vi "S Parameter VST Measurement.vi"(8 "error in":errorcluster, 9 "SPML Settings":T2={"VST Resource Name"="5842_0", "RFSG Port"="Port1", "RFmx Port"="Port2", "RF Out Switch"="2599_S8", "RF Out Connection"={"Common RFout"="COM0", "Port1 Incident"="NC0", "Port2 Incident"="NO0"}, "RF In Switch"="2597_S12", "RF In Connection"={"Common RFin"="COM", "Port1 Reference"="CH1", "Port1 Test"="CH2", "Port2 Reference"="CH4", "Port2 Test"="CH3"}, "RFSG attenuation mode"=enum."<None>", "RFSG Constant Attenuation (dB)"=0.0, "Save Calibration File at"=path "", "Short S1P"=path "", "Open S1P"=path "", "Load S1P"=path "", "Through Adapter S2P"=path ""}, 11 "Test Configuration":T1={"Action"=enum."Measure", "Power Level (dBm)"=0.0, "External Gain (dB)"=-6.0, "Frequency Sweep"={"Start Frequency (Hz)"=6000000000.0, "Stop Frequency (Hz)"=12000000000.0, "Step Size (Hz)"=100000000.0}, "Type of Stimulus"=enum."CW", "Pulse Width (s)"=0.0, "PRI (s)"=0.0, "IF Bandwidth (Hz)"=10000.0, "Average Mode"=enum."Per Sweep", "Number of Averages"=1, "SnP File Path"=path "", "Calibration File Path"=path "C:/Users/ies-pg-8881/Desktop/Andy/FPT/S_param_VST/S_param_cal_4.tdms"} {"Frequency Sweep"."Step Size (Hz)" format="%#_6p"; "Frequency Sweep"."Stop Frequency (Hz)" format="%.3p"; "Frequency Sweep"."Start Frequency (Hz)" format="%.3p"}) -> (0 "error out":errorcluster={"status"=TRUE, "code"=-1074134944, "source"="RFmxVNA Calibration Initiate.vi\r\n<ERR>IVI: (Hex 0xBFFA0060) Insufficient location information or resource not present in the system.  "}, 5 "S-Param Phase":dbl[][](array[numeric]), 7 "S-Param Magnitude":dbl[][](array[numeric]))   [LabVIEW 2023]
uses:
  Controls/Hardware Config - SParam_VST.ctl
  Controls/Test Config - SParam_VST.ctl
  <vilib>/niSPML/S-Parameter Measurements.lvlib
panel:
  out "SParam3":T3(graph)
  out "SParam1":T3(graph)
  out "SParam2":T3(graph)
  out "SParam0":T3(graph)
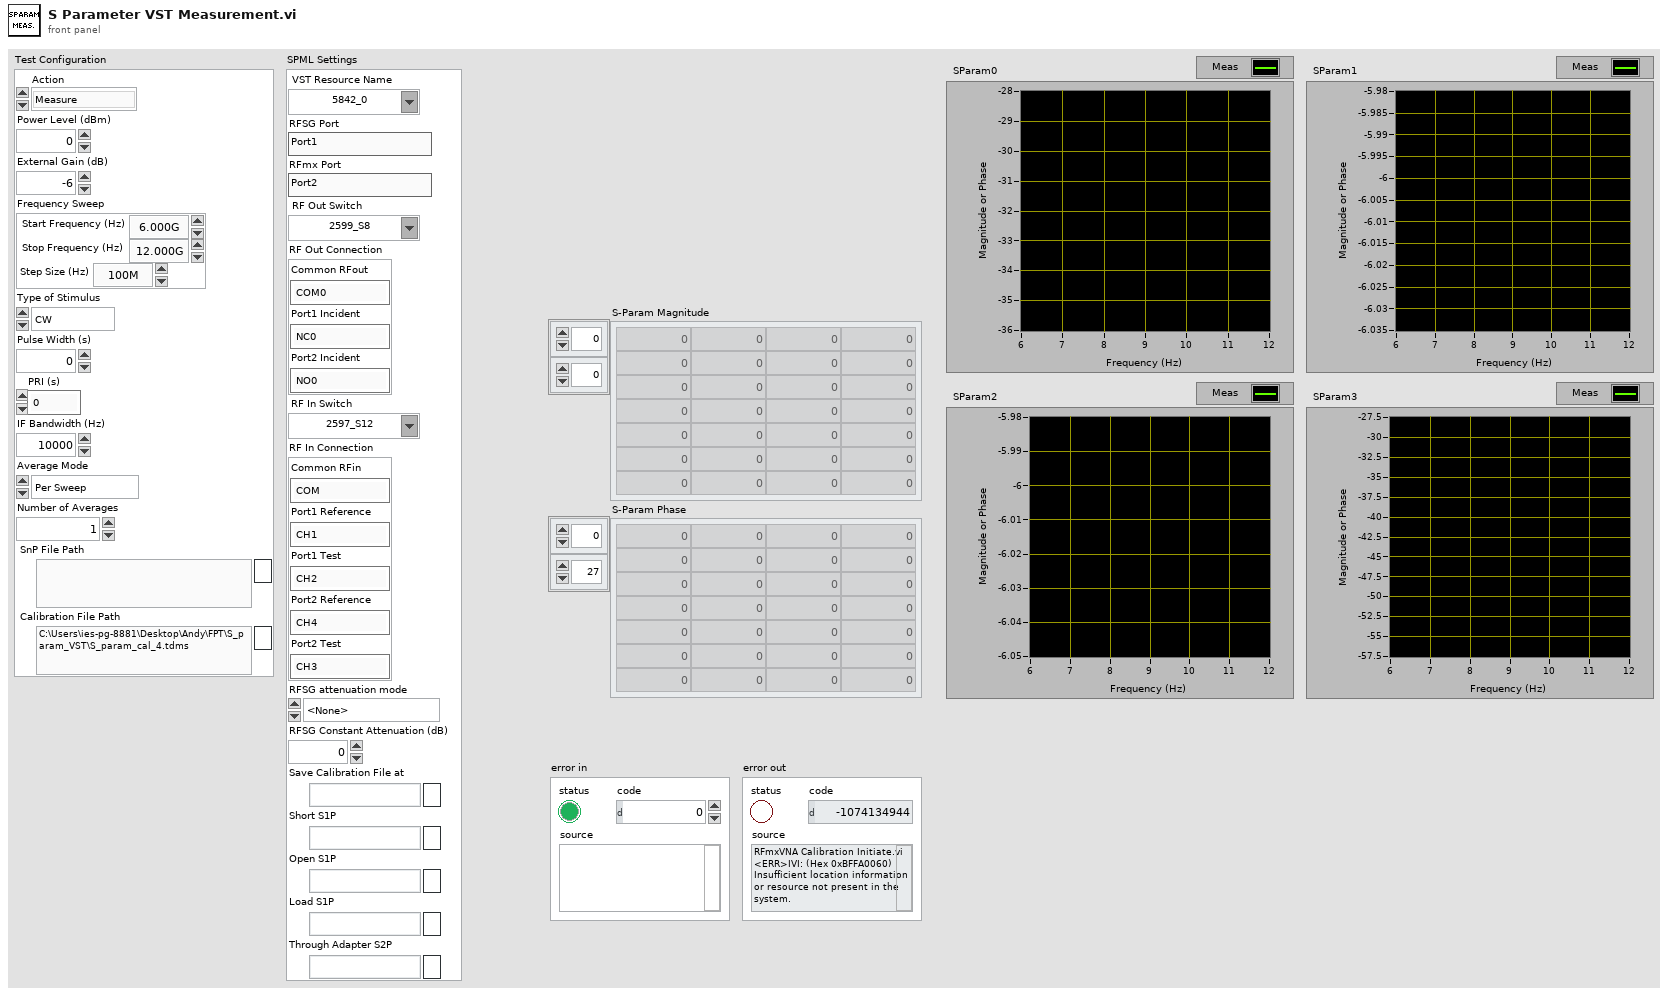
[diagram p1: front panel]
types:
  T1 = typedef "Test Config - SParam_VST.ctl" = cluster{"Action":enum32{"Calibrate", "Measure"}, "Power Level (dBm)":dbl, "External Gain (dB)":dbl, "Frequency Sweep":cluster{"Start Frequency (Hz)":dbl, "Stop Frequency (Hz)":dbl, "Step Size (Hz)":dbl}, "Type of Stimulus":enum16{"CW", "Pulsed CW"}, "Pulse Width (s)":dbl, "PRI (s)":dbl, "IF Bandwidth (Hz)":dbl, "Average Mode":enum16{"Per Sweep", "Per Point"}, "Number of Averages":i32, "SnP File Path":path, "Calibration File Path":path}
  T2 = typedef "Hardware Config - SParam_VST.ctl" = cluster{"VST Resource Name":refnum<k15>, "RFSG Port":string, "RFmx Port":string, "RF Out Switch":refnum<k15>, "RF Out Connection":cluster{"Common RFout":string, "Port1 Incident":string, "Port2 Incident":string}, "RF In Switch":refnum<k15>, "RF In Connection":cluster{"Common RFin":string, "Port1 Reference":string, "Port1 Test":string, "Port2 Reference":string, "Port2 Test":string}, "RFSG attenuation mode":enum32{"<None>", "Constant Attenuation"}, "RFSG Constant Attenuation (dB)":dbl, "Save Calibration File at":path, "Short S1P":path, "Open S1P":path, "Load S1P":path, "Through Adapter S2P":path}
  T3 = cluster{"S-Param Magnitude":dbl[], "S-Param Magnitude":dbl[]}
  T4 = typedef "S-Parameter Measurements.lvlib/S-Par Reference.lvclass/Session Handle.ctl" = refnum<data-value>
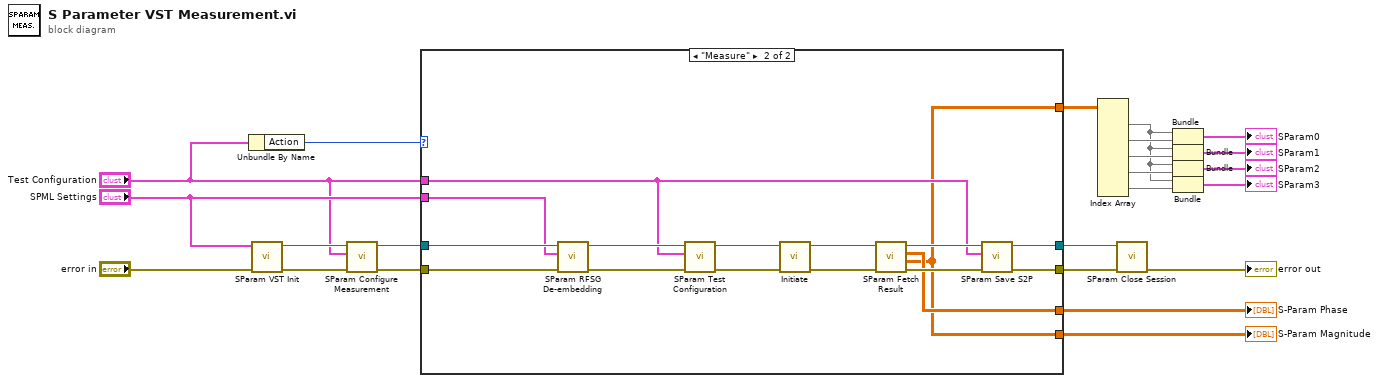
[diagram p0: block diagram]
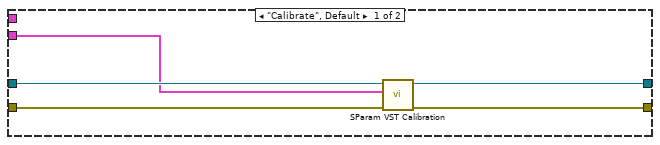
[diagram p2: hidden frame]
diagram:
  n1 = Unbundle By Name("Test Configuration") -> ("Action"=w22:enum32{"Calibrate", "Measure"})
  n2 = call "SParam VST Init.vi"("error in"="error in", "SPML Settings"="SPML Settings") -> ("error out"=w18:errorcluster, "S-Par Reference Out"=w17:T4)  [unwired: 8 in]
  n3 = call "SParam Configure Measurement.vi"("error in"=w18, "Test Configuration"="Test Configuration", "S-Par Reference In"=w17) -> ("error out"=w14:errorcluster, "S-Par Reference Out"=w15:T4)  [unwired: 7 in]
  n4 = case shown="\"Measure\"" w22 {
    tunnel: [_ w29] -> w13
    tunnel: [w25 w35] -> w3
    tunnel: [w24 w44] -> w2
    tunnel: w15 -> [w27 w40]
    tunnel: w14 -> [w28 w41]
    tunnel: "Test Configuration" -> [_ w31]
    tunnel: "SPML Settings" -> [w26 w32]
    tunnel: [_ w29] -> w21
    tunnel: [_ w30] -> w20
    frame "Calibrate", Default {
      n5 = call "SParam VST Calibration.vi"("error in"=w28, "RFmxVNA Settings"=w26, "S-Par Reference In"=w27) -> ("error out"=w24:errorcluster, "S-Par Reference Out"=w25:T4)  [unwired: 7 in]
    }
    frame "Measure" {
      n6 = call "SParam RFSG De-embedding.vi"("error in"=w41, "RFmxVNA Settings"=w32, "S-Par Reference In"=w40) -> ("error out"=w38:errorcluster, "S-Par Reference Out"=w39:T4)  [unwired: 7 in]
      n7 = call "SParam Test Configuration.vi"("error in"=w38, "Test Configuration"=w31, "S-Par Reference In"=w39) -> ("error out"=w36:errorcluster, "S-Par Reference Out"=w37:T4)  [unwired: 7 in]
      n8 = call <vilib>:"Initiate.vi"("S-Par Reference In"=w37, "error in"=w36) -> ("S-Par Reference Out"=w34:T4, "error out"=w33:errorcluster)  [unwired: 12 in]
      n9 = call "SParam Fetch Result.vi"("error in"=w33, "S-Par Reference In"=w34) -> ("error out"=w43:errorcluster, "S-Param Magnitude"=w29:dbl[][], "S-Param Phase"=w30:dbl[][], "S-Par Reference Out"=w42:T4)  [unwired: 6 in]
      n10 = call "SParam Save S2P.vi"("error in"=w43, "Test Configuration"=w31, "S-Par Reference In"=w42) -> ("error out"=w44:errorcluster, "S-Par Reference Out"=w35:T4)  [unwired: 7 in]
    }
  }
  "S-Param Magnitude" <- w21
  "S-Param Phase" <- w20
  n11 = Index Array(array=w13) -> (element #1=w8:dbl[], element #2=w9:dbl[], element #3=w10:dbl[], element #4=w11:dbl[], element #5=w12:dbl[])  [unwired: 10 in]
  n12 = call "SParam Close Session.vi"("error in"=w2, "S-Par Reference In"=w3) -> ("error out"=→"error out":errorcluster)  [unwired: 9 in]
  n13 = Bundle("S-Param Magnitude"=w8, "S-Param Magnitude"=w9) -> (→"SParam0":T3)  [unwired: 1 in]
  n14 = Bundle("S-Param Magnitude"=w8, "S-Param Magnitude"=w10) -> (→"SParam1":T3)  [unwired: 1 in]
  n15 = Bundle("S-Param Magnitude"=w8, "S-Param Magnitude"=w11) -> (→"SParam2":T3)  [unwired: 1 in]
  n16 = Bundle("S-Param Magnitude"=w8, "S-Param Magnitude"=w12) -> (→"SParam3":T3)  [unwired: 1 in]
